vi "HFRR ADV v05.vi"() -> ()   [LabVIEW 2025] (continued)
            n1941 = property on="XY Graph 13" class="XYGraph (strict)"("Y Scale.Display Format:Precision"=u8 0 ("Y Scale.Format & Precision:Precision")) -> ()  [unwired: 2 in, 2 out]
            n1942 = property on="XY Graph 13" class="XYGraph (strict)"("X Scale.Range:Minimum"=0.0, "X Scale.Range:Maximum"=75.0, "Y Scale.Range:Minimum"=0.0, "Y Scale.Range:Maximum"=100.0) -> ()  [unwired: 2 in, 2 out]
          }
        }
        n1943 = case shown="True" "RST CP" {
          frame False {
          }
          frame True {
            n1944 = property on="Sample Temperature" class="XYGraph (strict)"("Y Scale.Display Format:Precision"=u8 2 ("Y Scale.Format & Precision:Precision")) -> ()  [unwired: 2 in, 2 out]
            n1945 = property on="Sample Temperature" class="XYGraph (strict)"("X Scale.Range:Minimum"=0.0, "X Scale.Range:Maximum"=75.0, "Y Scale.Range:Minimum"=58.0, "Y Scale.Range:Maximum"=62.0) -> ()  [unwired: 2 in, 2 out]
          }
        }
        n1946 = case shown="True" "RSTV1 3" {
          frame False {
          }
          frame True {
            n1947 = property on="Air Temperature" class="XYGraph (strict)"("Y Scale.Display Format:Precision"=u8 2 ("Y Scale.Format & Precision:Precision")) -> ()  [unwired: 2 in, 2 out]
            n1948 = property on="Air Temperature" class="XYGraph (strict)"("X Scale.Range:Minimum"=0.0 ("Y Scale.Range:Minimum"), "X Scale.Range:Maximum"=75.0 ("Y Scale.Range:Maximum"), "Y Scale.Range:Minimum"=20.0 ("X Scale.Range:Minimum"), "Y Scale.Range:Maximum"=26.0 ("X Scale.Range:Maximum")) -> ()  [unwired: 2 in, 2 out]
          }
        }
        n1949 = case shown="True" "RSTV1 4" {
          frame False {
          }
          frame True {
            n1950 = property on="Stroke" class="XYGraph (strict)"("Y Scale.Display Format:Precision"=u8 2 ("Y Scale.Format & Precision:Precision")) -> ()  [unwired: 2 in, 2 out]
            n1951 = property on="Stroke" class="XYGraph (strict)"("X Scale.Range:Minimum"=0.0 ("Y Scale.Range:Maximum"), "X Scale.Range:Maximum"=75.0 ("X Scale.Range:Minimum"), "Y Scale.Range:Minimum"=0.98, "Y Scale.Range:Maximum"=1.02) -> ()  [unwired: 2 in, 2 out]
          }
        }
        n1952 = case shown="True" "rstv2" {
          frame False {
          }
          frame True {
            n1953 = property on="Coefficient Of Friction" class="XYGraph (strict)"("Y Scale.Display Format:Precision"=u8 3 ("Y Scale.Format & Precision:Precision")) -> ()  [unwired: 2 in, 2 out]
            n1954 = property on="Coefficient Of Friction" class="XYGraph (strict)"("X Scale.Range:Minimum"=0.0 ("Y Scale.Range:Maximum"), "X Scale.Range:Maximum"=75.0, "Y Scale.Range:Minimum"=0.0, "Y Scale.Range:Maximum"=1.0 ("X Scale.Range:Minimum")) -> ()  [unwired: 2 in, 2 out]
          }
        }
        n1955 = case shown="True" "RST CP 3" {
          frame False {
          }
          frame True {
            n1956 = property on="Air Temp vs Rh" class="XYGraph (strict)"("X Scale.Range:Minimum"=18.0, "X Scale.Range:Maximum"=28.0 ("X Scale.Range:Minimum"), "Y Scale.Range:Minimum"=30.0 ("X Scale.Range:Minimum"), "Y Scale.Range:Maximum"=70.0 ("X Scale.Range:Minimum")) -> ()  [unwired: 2 in, 2 out]
          }
        }
        n1957 = case shown="True" "OPEN 1" {
          frame False {
          }
          frame True {
            (unwired) 0  # existing file
            w2822 = "Choose a datalog file to open"  # prompt
            n1958 = local write "OPEN 1"(FALSE ("OPEN 1")) -> ()
            n1959 = String To Path(string="C:\\LAB-IQ-NXT\\Data\\") -> (path=w2807:path)
            n1960 = File Dialog(6:"*.dgf" ("pattern"), 7:w2822, 11:w2807) -> (0:w2805:errorcluster, 3:w2813:path)  [unwired: 4 in, 2 out]
            n1961 = Unbundle(w2805) -> ()  [unwired: 3 out]
            n1962 = Strip Path(path=w2813) -> (name=w2812:string)  [unwired: 1 out]
            n1963 = Path To String(path=w2813) -> (string=w2808:string)
            "string1" <- w2808
            n1964 = Match Pattern(string=w2812, regular expression=".dgf") -> (before substring=→"String Control":string)  [unwired: 1 in, 3 out]
            n1965 = Match Pattern(string=w2808, regular expression=".dgf" ("substring (\"\")")) -> (before substring=w2818:string)  [unwired: 1 in, 3 out]
            n1966 = Concatenate Strings(w2818, ".duf" ("Substring")) -> (w2814:string)
            n1967 = String To Path(string=w2814) -> (path=w2819:path)
            n1968 = call <vilib>:"Read Characters From File.vi"("file path (dialog if empty)"=w2819, "start of read offset (chars.:0)"=60 ("start of read offset (chars.: 0)")) -> ("character string"=→"String Control 2":string)  [unwired: 4 in, 3 out]
          }
        }
        n1969 = case shown="True" "OPEN 2" {
          frame False {
          }
          frame True {
            (unwired) 0  # existing file
            w2840 = "Choose a datalog file to open"  # prompt
            n1970 = local write "OPEN 2"(FALSE ("OPEN 1")) -> ()
            n1971 = String To Path(string="C:\\LAB-IQ-NXT\\Data\\") -> (path=w2825:path)
            n1972 = File Dialog(6:"*.dgf" ("pattern"), 7:w2840, 11:w2825) -> (0:w2823:errorcluster, 3:w2831:path)  [unwired: 4 in, 2 out]
            n1973 = Unbundle(w2823) -> ()  [unwired: 3 out]
            n1974 = Strip Path(path=w2831) -> (name=w2829:string)  [unwired: 1 out]
            n1975 = Path To String(path=w2831) -> (string=w2826:string)
            "string1 2" <- w2826
            n1976 = Match Pattern(string=w2829, regular expression=".dgf") -> (before substring=→"String Control 3":string)  [unwired: 1 in, 3 out]
            n1977 = Match Pattern(string=w2826, regular expression=".dgf" ("substring (\"\")")) -> (before substring=w2837:string)  [unwired: 1 in, 3 out]
            n1978 = Concatenate Strings(w2837, ".duf" ("Substring")) -> (w2834:string)
            n1979 = String To Path(string=w2834) -> (path=w2832:path)
            n1980 = call <vilib>:"Read Characters From File.vi"("file path (dialog if empty)"=w2832, "start of read offset (chars.:0)"=60 ("start of read offset (chars.: 0)")) -> ("character string"=→"String Control 4":string)  [unwired: 4 in, 3 out]
          }
        }
        n1981 = case shown="True" "OPEN 3" {
          frame False {
          }
          frame True {
            (unwired) 0  # existing file
            w2858 = "Choose a datalog file to open"  # prompt
            n1982 = local write "OPEN 3"(FALSE ("OPEN 1")) -> ()
            n1983 = String To Path(string="C:\\LAB-IQ-NXT\\Data\\") -> (path=w2843:path)
            n1984 = File Dialog(6:"*.dgf" ("pattern"), 7:w2858, 11:w2843) -> (0:w2841:errorcluster, 3:w2849:path)  [unwired: 4 in, 2 out]
            n1985 = Unbundle(w2841) -> ()  [unwired: 3 out]
            n1986 = Strip Path(path=w2849) -> (name=w2847:string)  [unwired: 1 out]
            n1987 = Path To String(path=w2849) -> (string=w2844:string)
            "string1 3" <- w2844
            n1988 = Match Pattern(string=w2847, regular expression=".dgf") -> (before substring=→"String Control 5":string)  [unwired: 1 in, 3 out]
            n1989 = Match Pattern(string=w2844, regular expression=".dgf" ("substring (\"\")")) -> (before substring=w2854:string)  [unwired: 1 in, 3 out]
            n1990 = Concatenate Strings(w2854, ".duf" ("Substring")) -> (w2851:string)
            n1991 = String To Path(string=w2851) -> (path=w2855:path)
            n1992 = call <vilib>:"Read Characters From File.vi"("file path (dialog if empty)"=w2855, "start of read offset (chars.:0)"=60 ("start of read offset (chars.: 0)")) -> ("character string"=→"String Control 6":string)  [unwired: 4 in, 3 out]
          }
        }
        n1993 = case shown="True" "OPEN 4" {
          frame False {
          }
          frame True {
            (unwired) 0  # existing file
            w2876 = "Choose a datalog file to open"  # prompt
            n1994 = local write "OPEN 4"(FALSE ("OPEN 1")) -> ()
            n1995 = String To Path(string="C:\\LAB-IQ-NXT\\Data\\") -> (path=w2861:path)
            n1996 = File Dialog(6:"*.dgf" ("pattern"), 7:w2876, 11:w2861) -> (0:w2859:errorcluster, 3:w2867:path)  [unwired: 4 in, 2 out]
            n1997 = Unbundle(w2859) -> ()  [unwired: 3 out]
            n1998 = Strip Path(path=w2867) -> (name=w2865:string)  [unwired: 1 out]
            n1999 = Path To String(path=w2867) -> (string=w2862:string)
            "string1 4" <- w2862
            n2000 = Match Pattern(string=w2865, regular expression=".dgf") -> (before substring=→"String Control 7":string)  [unwired: 1 in, 3 out]
            n2001 = Match Pattern(string=w2862, regular expression=".dgf" ("substring (\"\")")) -> (before substring=w2872:string)  [unwired: 1 in, 3 out]
            n2002 = Concatenate Strings(w2872, ".duf" ("Substring")) -> (w2869:string)
            n2003 = String To Path(string=w2869) -> (path=w2873:path)
            n2004 = call <vilib>:"Read Characters From File.vi"("file path (dialog if empty)"=w2873, "start of read offset (chars.:0)"=60 ("start of read offset (chars.: 0)")) -> ("character string"=→"String Control 8":string)  [unwired: 4 in, 3 out]
          }
        }
      }
      frame "About" {
        # "Elapsed time\ncof\nstroke\nmean pos\nTemp\nHumidity"
        n2005 = disable-structure shown="Disabled" {
          frame Disabled {
            n2006 = case shown="True" "Export" {
              frame False {
              }
              frame True {
                w2898 = "                                      " ("string")
                w2900 = "\r"
                (unwired) i16 6 ("width (-)")
                w2977 = "\r"
                w2909 = "\r"
                n2007 = local write "Export"(FALSE ("Export")) -> ()
                n2008 = local read "String 29"() -> (w2946:string)
                n2009 = local read "String 34"() -> (w2934:string)
                n2010 = local read "String 35"() -> (w2929:string)
                n2011 = local read "String 37"() -> (w2925:string)
                n2012 = local read "String 36"() -> (w2922:string)
                n2013 = local read "String 38"() -> (w2919:string)
                n2014 = local read "String 39"() -> (w2916:string)
                n2015 = Match Pattern(string=w2946, regular expression=".dwm") -> (before substring=w2942:string)  [unwired: 1 in, 3 out]
                "before substring" <- w2942
                n2016 = local read "S 38"() -> (w2937:string)
                n2017 = local read "S 39"() -> (w2930:string)
                n2018 = local read "Temperature before test 2"() -> (w2966:dbl)
                n2019 = local read "Temperature after test 2"() -> (w2971:dbl)
                n2020 = local read "Humidity before test 2"() -> (w2952:dbl)
                n2021 = local read "Humidity after test 2"() -> (w2967:dbl)
                n2022 = local read "MWSD 2"() -> (w2963:dbl)
                n2023 = local read "WS1.4 2"() -> (w2979:dbl)
                n2024 = local read "HCF 2"() -> (w2975:dbl)
                n2025 = local read "AVP 2"() -> (w2964:dbl)
                n2026 = Concatenate Strings("1," ("string"), w2937) -> (w2936:string)
                n2027 = Concatenate Strings("2," ("string"), w2934) -> (w2933:string)
                n2028 = Concatenate Strings("3," ("string"), w2930) -> (w2932:string)
                n2029 = Concatenate Strings("4," ("string"), w2929) -> (w2928:string)
                n2030 = Concatenate Strings("5," ("string"), w2925) -> (w2926:string)
                n2031 = Concatenate Strings("6," ("string"), w2922) -> (w2923:string)
                n2032 = Concatenate Strings("7," ("string"), w2919) -> (w2920:string)
                n2033 = Concatenate Strings("8," ("string"), w2916) -> (w2917:string)
                n2034 = local read "Sample ID"() -> (w2984:string)
                n2035 = case shown="\"xlx\"" "Select File Type" {
                  tunnel: w2942 -> [w2987 w2989 w2991]
                  tunnel: [w2985 w2990 w2992] -> w2941
                  frame "xlx" {
                    n2036 = Concatenate Strings(w2987, ".xls" ("string")) -> (w2985:string)
                  }
                  frame "csv" {
                    n2037 = Concatenate Strings(w2989, ".csv" ("string")) -> (w2990:string)
                  }
                  frame "txt" {
                    n2038 = Concatenate Strings(w2991, ".txt" ("string")) -> (w2992:string)
                  }
                }
                n2039 = local read "Test Date"() -> (w2983:string)
                n2040 = local read "String 45"() -> (w2897:string)
                n2041 = local read "String 31"() -> (w2982:string)
                n2042 = local read "String 32"() -> (w2981:string)
                n2043 = local read "TITTLE"() -> (w2905:string)
                n2044 = Number To Fractional String(number=w2952, width (-)=i16 6, precision (6)=i16 2) -> (F-format string=w2951:string)  [unwired: 1 in]
                n2045 = Number To Fractional String(number=w2966, width (-)=i16 6, precision (6)=i16 2) -> (F-format string=w2972:string)  [unwired: 1 in]
                n2046 = Number To Fractional String(number=w2967, width (-)=i16 6, precision (6)=i16 2) -> (F-format string=w2965:string)  [unwired: 1 in]
                n2047 = Number To Fractional String(number=w2971, width (-)=i16 6, precision (6)=i16 2) -> (F-format string=w2970:string)  [unwired: 1 in]
                n2048 = Number To Fractional String(number=w2963, width (-)=i16 6, precision (6)=i16 2) -> (F-format string=w2961:string)  [unwired: 1 in]
                n2049 = Number To Fractional String(number=w2964, width (-)=i16 6, precision (6)=i16 2) -> (F-format string=w2962:string)  [unwired: 1 in]
                n2050 = Number To Fractional String(number=w2975, width (-)=i16 6, precision (6)=i16 2) -> (F-format string=w2976:string)  [unwired: 1 in]
                n2051 = Number To Fractional String(number=w2979, precision (6)=i16 2) -> (F-format string=w2980:string)  [unwired: 2 in]
                n2052 = local read "s.NO"() -> (w2899:string)
                n2053 = Concatenate Strings("=" ("string"), w2905) -> (w2904:string)
                n2054 = Concatenate Strings("S.No," ("string"), "                                       Parameters" ("string")) -> (w2910:string)
                n2055 = Concatenate Strings(w2977, w2936, w2951, w2977, w2933, w2972, w2977, w2932, w2965, w2977, w2928, w2970, w2977, w2926, w2961, w2977, w2923, w2962, w2977, w2920, w2976, w2977, w2917, w2980) -> (w2939:string)
                n2056 = Concatenate Strings(w2909, "," ("string"), w2897, w2899, w2898, w2981, w2984, w2898, w2982, w2983, w2909) -> (w2907:string)
                n2057 = local read "Tested by"() -> (w2913:string)
                n2058 = local read "String 33"() -> (w2914:string)
                n2059 = Concatenate Strings("," ("string"), "                                                                             " ("string")) -> (w2902:string)
                n2060 = Concatenate Strings(w2904, w2900, w2907, w2900, w2910, w2939, w2900, w2902, w2914, w2913) -> (→"export":string)
                n2061 = String To Path(string=w2941) -> (path=w2948:path)
                n2062 = local read "export"() -> (w2943:string)
                n2063 = call <vilib>:"Write Characters To File.vi"("append to file? (new file:F)"=FALSE, "character string"=w2943, "file path (dialog if empty)"=w2948) -> ()  [unwired: 2 in, 1 out]
              }
            }
          }
          frame Enabled {
          }
        }
        n2064 = case shown="True" "OK Button 17" {
          frame False {
          }
          frame True {
            (unwired) 0  # existing file
            w3201 = "Choose a datalog file to open"  # prompt
            n2065 = local write "OK Button 17"(FALSE ("OK Button 17")) -> ()
            n2066 = local read "String"() -> (w3196:string)
            n2067 = String To Path(string=w3196) -> (path=w3197:path)
            n2068 = File Dialog(6:"*.duf" ("pattern"), 7:w3201, 11:w3197) -> (0:w3188:errorcluster, 3:w3207:path)  [unwired: 4 in, 2 out]
            n2069 = Unbundle(w3188) -> ()  [unwired: 3 out]
            n2070 = Open/Create/Replace File "Open File"(file path (use dialog)=w3207) -> (refnum out=w3199:refnum<file>)  [unwired: 5 in, 2 out]
            n2071 = Strip Path(path=w3207) -> (name=w3205:string)  [unwired: 1 out]
            n2072 = Path To String(path=w3207) -> (string=w3190:string)
            n2073 = while {
              tunnel: w3199 -> [w3211]
              i -> [w3208]
              stop <- w3209 continue-if-true
              (unwired) TRUE ("line mode (F)")
              n2074 = Read from Text File "Read File"(file (use dialog)=w3211) -> (text=w3210:string)  [unwired: 3 in, 3 out]
              n2075 = local write "Numeric 16"(w3208) -> ()
              n2076 = String Length(string=w3210) -> (length=w3213:i32)
              n2077 = Greater?(x=w3213, y=1) -> (0:w3209:bool)
            }
            n2078 = local write "String 29"(w3190) -> ()
            n2079 = Search and Replace String(input string=w3190, search string=".duf", replace string=".dgf" ("replace string (\"\")")) -> (result string=→"String Indicator 4":string)  [unwired: 5 in, 3 out]
            n2080 = Match Pattern(string=w3205, regular expression=".dwm") -> (before substring=w3189:string)  [unwired: 1 in, 3 out]
            "String Indicator" <- w3189
            n2081 = Match Pattern(string=w3190, regular expression=".dwm" ("substring (\"\")")) -> (before substring=w3191:string)  [unwired: 1 in, 3 out]
            "String Indicator 3" <- w3191
            n2082 = local write "TITTLE 2"(w3189) -> ()
            n2083 = String To Path(string=w3191) -> (path=w3198:path)
            "path" <- w3198
            n2084 = call <vilib>:"Read Characters From File.vi"("file path (dialog if empty)"=w3198, "start of read offset (chars.:0)"=60 ("start of read offset (chars.: 0)")) -> ("character string"=→"String Indicator 2":string)  [unwired: 4 in, 3 out]
          }
        }
        n2085 = case shown="True" "OK Button 16" {
          frame False {
          }
          frame True {
            n2086 = stacked-sequence {
              frame #0 {
                n2087 = local read "Numeric 16"() -> (w3215:i32)
                n2088 = local write "Numeric 10"(w3215) -> ()
              }
              frame #1 {
                n2089 = local read "S.NO"() -> (→"s.NO":string)
                n2090 = local read "String 29"() -> (w3219:string)
                n2091 = String To Path(string=w3219) -> (path=w3218:path)
                n2092 = Open/Create/Replace File "Open File"(file path (use dialog)=w3218) -> (refnum out=w3220:refnum<file>)  [unwired: 5 in, 2 out]
                n2093 = for {
                  N: 16 -> [_]
                  tunnel: w3220 -> [w3227]
                  i -> [w3223]
                  (unwired) TRUE ("line mode (F)")
                  n2094 = Read from Text File "Read File"(file (use dialog)=w3227) -> (text=w3221:string)  [unwired: 3 in, 3 out]
                  n2095 = Match Pattern(string=w3221, regular expression="(") -> (after substring=w3226:string)  [unwired: 1 in, 3 out]
                  n2096 = Match Pattern(string=w3226, regular expression=")") -> (before substring=w3222:string)  [unwired: 1 in, 3 out]
                  n2097 = case shown="1" w3223 {
                    tunnel: w3222 -> [w3228 w3229 _ _ w3230 w3231 w3232 w3234 w3236 w3238 w3240 w3242 w3244 w3246 _]
                    tunnel: w3221 -> [_ _ _ _ _ _ _ _ _ _ _ _ _ _ _]
                    frame 0 {
                      "TITTLE" <- w3228
                    }
                    frame 1 {
                      "Sample ID" <- w3229
                    }
                    frame 2 {
                    }
                    frame 3 {
                    }
                    frame 4 {
                      "Test Date" <- w3230
                    }
                    frame 5 {
                      "Tested by" <- w3231
                    }
                    frame 6 {
                      n2098 = Fract/Exp String To Number(string=w3232) -> (number=→"Humidity before test 2":dbl)  [unwired: 3 in, 1 out]
                    }
                    frame 7 {
                      n2099 = Fract/Exp String To Number(string=w3234) -> (number=→"Temperature before test 2":dbl)  [unwired: 3 in, 1 out]
                    }
                    frame 8 {
                      n2100 = Fract/Exp String To Number(string=w3236) -> (number=→"Humidity after test 2":dbl)  [unwired: 3 in, 1 out]
                    }
                    frame 9 {
                      n2101 = Fract/Exp String To Number(string=w3238) -> (number=→"Temperature after test 2":dbl)  [unwired: 3 in, 1 out]
                    }
                    frame 10 {
                      n2102 = Fract/Exp String To Number(string=w3240) -> (number=→"MWSD 2":dbl)  [unwired: 3 in, 1 out]
                    }
                    frame 11 {
                      n2103 = Fract/Exp String To Number(string=w3242) -> (number=→"AVP 2":dbl)  [unwired: 3 in, 1 out]
                    }
                    frame 12 {
                      n2104 = Fract/Exp String To Number(string=w3244) -> (number=→"HCF 2":dbl)  [unwired: 3 in, 1 out]
                    }
                    frame 13 {
                      n2105 = Fract/Exp String To Number(string=w3246) -> (number=→"WS1.4 2":dbl)  [unwired: 3 in, 1 out]
                    }
                    frame 14, Default {
                    }
                  }
                }
              }
              frame #2 {
              }
            }
            n2106 = local write "OK Button 16"(FALSE ("OK Button 13")) -> ()
          }
        }
        n2107 = call <vilib>:"Query Available Printers.vi"() -> ("system configured printers"=w2890:string[])  [unwired: 9 in, 2 out]
        "System Configured Printers 2" <- w2890
        n2108 = local read "OK Button 16"() -> (w2887:bool)
        n2109 = Index Array(array=w2890, index="Select Printer 3") -> (element=w2892:string)
        "Selected Printer" <- w2892
        n2110 = case shown="True" w2887 {
          frame False {
          }
          frame True {
            n2111 = flat-sequence {
              frame #0 {
              }
              frame #1 {
                n2112 = Wait (ms)(milliseconds to wait=u32 100) -> ()  [unwired: 1 out]
              }
              frame #2 {
                n2113 = local write "OK Button 16"(FALSE ("Print 3")) -> ()
              }
            }
          }
        }
        n2114 = case shown="True" "Print" {
          tunnel: w2892 -> [_ w3184]
          frame False {
          }
          frame True {
            (unwired) i16 6 ("width (-)")
            (unwired) "TESTED BY : "
            (unwired) "TESTED DATE :"
            (unwired) "SAMPLE ID : "
            (unwired) "SAMPLE DESIGN : "
            w3142 = "\r"
            w3159 = "\r"
            # "add image"
            n2115 = local read "Sample ID"() -> (w3132:string)
            n2116 = local read "Tested by"() -> (w3135:string)
            n2117 = local read "String 34"() -> (w3122:string)
            n2118 = local read "String 45"() -> (w3102:string)
            n2119 = local read "String 35"() -> (w3117:string)
            n2120 = local read "String 37"() -> (w3115:string)
            n2121 = local read "String 32"() -> (w3137:string)
            n2122 = local read "String 36"() -> (w3112:string)
            n2123 = local read "String 31"() -> (w3136:string)
            n2124 = local read "Test Date"() -> (w3133:string)
            n2125 = local read "String 33"() -> (w3138:string)
            n2126 = local read "String 38"() -> (w3108:string)
            n2127 = local read "String 39"() -> (w3105:string)
            n2128 = local write "Print"(FALSE ("Print FF")) -> ()
            n2129 = local read "S 39"() -> (w3120:string)
            n2130 = local read "S 38"() -> (w3127:string)
            n2131 = local read "Temperature before test 2"() -> (w3158:dbl)
            n2132 = local read "Temperature after test 2"() -> (w3148:dbl)
            n2133 = local read "Humidity before test 2"() -> (w3173:dbl)
            n2134 = local read "Humidity after test 2"() -> (w3157:dbl)
            n2135 = local read "MWSD 2"() -> (w3162:dbl)
            n2136 = local read "WS1.4 2"() -> (w3140:dbl)
            n2137 = Concatenate Strings("2)" ("string"), w3122) -> (w3123:string)
            n2138 = Concatenate Strings("3)" ("string"), w3120) -> (w3121:string)
            n2139 = Concatenate Strings("1)" ("string"), w3127) -> (w3126:string)
            n2140 = Concatenate Strings("4)" ("string"), w3117) -> (w3118:string)
            n2141 = Concatenate Strings("5)" ("string"), w3115) -> (w3114:string)
            n2142 = Concatenate Strings("6)" ("string"), w3112) -> (w3111:string)
            n2143 = Concatenate Strings("7)" ("string"), w3108) -> (w3109:string)
            n2144 = Concatenate Strings("8)" ("string"), w3105) -> (w3106:string)
            n2145 = local read "HCF 2"() -> (w3144:dbl)
            n2146 = local read "AVP 2"() -> (w3161:dbl)
            n2147 = local read "s.NO"() -> (w3103:string)
            n2148 = call <vilib>:"New Report.vi"("report type"=enum16{"Standard Report", "HTML"}."Standard Report") -> ("report out"=w3182:refnum<class "NI_report.lvclass">, "error out"=w3181:errorcluster)  [unwired: 13 in]
            n2149 = local read "TITTLE"() -> (w3134:string)
            n2150 = Concatenate Strings(w3159, w3102, w3103, w3159, w3137, w3132, w3159, w3136, w3133, w3159, w3138, w3135, w3159) -> (w3152:string)
            "test by" <- w3152
            n2151 = Number To Fractional String(number=w3158, width (-)=i16 6, precision (6)=i16 2) -> (F-format string=w3147:string)  [unwired: 1 in]
            n2152 = Number To Fractional String(number=w3157, width (-)=i16 6, precision (6)=i16 2) -> (F-format string=w3160:string)  [unwired: 1 in]
            n2153 = Number To Fractional String(number=w3173, width (-)=i16 6, precision (6)=i16 2) -> (F-format string=w3178:string)  [unwired: 1 in]
            n2154 = Number To Fractional String(number=w3162, width (-)=i16 6, precision (6)=i16 2) -> (F-format string=w3164:string)  [unwired: 1 in]
            n2155 = Number To Fractional String(number=w3148, width (-)=i16 6, precision (6)=i16 2) -> (F-format string=w3149:string)  [unwired: 1 in]
            n2156 = Number To Fractional String(number=w3161, width (-)=i16 6, precision (6)=i16 2) -> (F-format string=w3163:string)  [unwired: 1 in]
            n2157 = Number To Fractional String(number=w3144, width (-)=i16 6, precision (6)=i16 2) -> (F-format string=w3143:string)  [unwired: 1 in]
            n2158 = Number To Fractional String(number=w3140, precision (6)=i16 2) -> (F-format string=w3139:string)  [unwired: 2 in]
            n2159 = call-dynamic "Set Report Header Text.vi"("report in"=w3182, "center header text"=w3134, "error in (no error)"=w3181) -> ("report out"=w3153:refnum<class "NI_report.lvclass">, "error out"=w3154:errorcluster)  [unwired: 11 in]
            n2160 = Concatenate Strings(w3142, w3126, w3178, w3142, w3123, w3147, w3142, w3121, w3160, w3142, w3118, w3149, w3142, w3114, w3164, w3142, w3111, w3163, w3142, w3109, w3143, w3142, w3106, w3139) -> (w3130:string)
            "export 2" <- w3130
            n2161 = call-poly <vilib>:"Append Report Text.vi"("report in"=w3153, "text"=w3152, "error in (no error)"=w3154) -> ("report out"=w3156:refnum<class "NI_report.lvclass">, "error out"=w3155:errorcluster)  [unwired: 9 in, 2 out]
            n2162 = local read "test by"() -> (w3129:string)
            n2163 = local read "TITTLE"() -> (w3131:string)
            n2164 = call-poly <vilib>:"Append Report Text.vi"("report in"=w3156, "error in (no error)"=w3155) -> ("report out"=w3177:refnum<class "NI_report.lvclass">, "error out"=w3175:errorcluster)  [unwired: 10 in, 2 out]
            n2165 = Concatenate Strings(w3131, w3130, w3129) -> (→"output":string)
            n2166 = call-poly <vilib>:"Append Report Text.vi"("report in"=w3177, "text"=w3130, "error in (no error)"=w3175) -> ("report out"=w3176:refnum<class "NI_report.lvclass">, "error out"=w3174:errorcluster)  [unwired: 9 in, 2 out]
            n2167 = call-dynamic "Print Report.vi"("report in"=w3176, "printer name (default)"=w3184, "error in (no error)"=w3174) -> ("report out"=w3186:refnum<class "NI_report.lvclass">, "error out"=w3187:errorcluster)  [unwired: 11 in]
            n2168 = call-dynamic "Dispose Report.vi"("report in"=w3186, "error in (no error)"=w3187) -> ()  [unwired: 13 in, 1 out]
          }
        }
        n2169 = case shown="True" "Print 2" {
          frame False {
          }
          frame True {
            n2170 = flat-sequence {
              frame #0 {
                n2171 = local read "s.NO"() -> (→"s.NO 2":string)
                n2172 = Wait (ms)(milliseconds to wait=u32 20) -> ()  [unwired: 1 out]
                n2173 = local read "Sample ID  3"() -> (→"Sample ID  6":string)
                n2174 = local read "Sample ID  4"() -> (→"Sample ID  7":string)
                n2175 = local read "Sample ID"() -> (→"Sample ID  2":string)
                n2176 = local read "Tested by"() -> (→"Tested by 2":string)
                n2177 = local read "Test Date"() -> (→"Test Date 2":string)
                n2178 = local read "Humidity after test 3"() -> (→"Humidity after test 4":dbl)
                n2179 = local read "Ref A Test Date :"() -> (→"TITTLE 4":string)
                n2180 = local read "Temperature before test 3"() -> (w3009:dbl)
                n2181 = local read "Temperature before test 3"() -> (→"Temperature after test 5":dbl)
                n2182 = local read "Temperature after test 3"() -> (→"Temperature after test 4":dbl)
                n2183 = local read "Humidity before test 3"() -> (→"Humidity before test 4":dbl)
                n2184 = local write "Temperature before test 3"(w3009) -> ()
                n2185 = local read "image data"() -> (w3000:T11)
                n2186 = String To Path(string="C:\\LAB-IQ-NXT\\im\\Temp_resized.jpg") -> (path=w3001:path)
                "path 2" <- w3001
                n2187 = call <vilib>:"Write JPEG File.vi"("image data"=w3000, "path to JPEG file"=w3001) -> ()  [unwired: 8 in, 2 out]
                "Ref A Test Date :" <- "Ref A Test Date :"
                "Ref B Test Date :" <- "Ref B Test Date :"
                "Ref B Scar Value :" <- "Ref B Scar Value :"
                "Ref A Scar Value :" <- "Ref A Scar Value :"
              }
              frame #1 {
                (unwired) HTML_Report_Image_Alignment."MIDDLE" ("alignment (default)")
                w3037 = u16 0 items=["portrait", "landscape"] ("orientation (portrait)")
                (unwired) HTML_Report_Image_Alignment."ABSMIDDLE" ("alignment (default)")
                (unwired) "TESTED BY : "
                (unwired) "TESTED DATE :"
                (unwired) "SAMPLE ID : "
                (unwired) "SAMPLE DESIGN : "
                w3070 = "\r"
                # "add image"
                n2188 = Wait (ms)(milliseconds to wait=u32 20) -> ()  [unwired: 1 out]
                n2189 = local read "Sample ID  2"() -> (w3063:string)
                n2190 = local read "Wear Scar X"() -> (w3035:dbl)
                "Length ( microns ) 2" <- w3035
                n2191 = local read "Wear Scar Y"() -> (w3034:dbl)
                "Wear Scar Y ( microns ) :" <- w3034
                n2192 = local read "Test Date 2"() -> (w3064:string)
                n2193 = local read "Tested by 2"() -> (w3065:string)
                n2194 = local read "String 46"() -> (w3061:string)
                n2195 = local read "String 48"() -> (w3067:string)
                n2196 = local read "String 47"() -> (w3066:string)
                n2197 = local read "String 49"() -> (w3068:string)
                n2198 = local read "String 10"() -> (w3021:string)
                n2199 = local read "s.NO 2"() -> (w3062:string)
                n2200 = Add(x=w3035, y=w3034) -> (x+y=w3033:dbl)
                n2201 = call <vilib>:"New Report.vi"("report type"=enum16{"Standard Report", "HTML"}."HTML") -> ("report out"=w3041:refnum<class "NI_report.lvclass">, "error out"=w3039:errorcluster)  [unwired: 13 in]
                n2202 = Concatenate Strings(w3070, w3061, w3062, w3070, w3067, w3063, w3070, w3066, w3064, w3070, w3068, w3065, w3070) -> (→"test by 2":string)
                n2203 = Concatenate Strings("C:\\LAB-IQ-NXT\\Data\\" ("string"), w3021, ".jpg" ("string")) -> ()  [unwired: 1 out]
                n2204 = Divide(x=w3033, y=2.0) -> (x/y=→"Mean Wear ( microns) :":dbl)
                n2205 = call-dynamic "Set Report Orientation.vi"("report in"=w3041, "orientation (portrait)"=w3037, "error in (no error)"=w3039) -> ("report out"=w3040:refnum<class "NI_report.lvclass">, "error out"=w3038:errorcluster)  [unwired: 11 in]
                n2206 = for {
                  N: 5 -> [_]
                  tunnel: w3040 -> [w3091]
                  tunnel: [w3090] -> w3019
                  tunnel: w3038 -> [w3089]
                  tunnel: [w3088] -> w3018
                  n2207 = call-dynamic "Set Report Tab Width.vi"("report in"=w3091, "error in (no error)"=w3089) -> ("report out"=w3090:refnum<class "NI_report.lvclass">, "error out"=w3088:errorcluster)  [unwired: 12 in]
                }
                n2208 = local read "TITTLE"() -> (w3036:string)
                n2209 = call-dynamic "Set Report Header Text.vi"("report in"=w3019, "center header text"=w3036, "error in (no error)"=w3018) -> ("report out"=w3057:refnum<class "NI_report.lvclass">, "error out"=w3056:errorcluster)  [unwired: 11 in]
                n2210 = for {
                  N: 1 -> [_]
                  tunnel: [w3095] -> w3043
                  tunnel: [w3094] -> w3042
                  tunnel: w3057 -> [w3093]
                  tunnel: w3056 -> [w3092]
                  n2211 = call-dynamic "New Report Line.vi"("report in"=w3093, "error in (no error)"=w3092) -> ("report out"=w3095:refnum<class "NI_report.lvclass">, "error out"=w3094:errorcluster)  [unwired: 12 in]
                }
                n2212 = for {
                  N: 2 -> [_]
                  tunnel: [w3087] -> w3049
                  tunnel: [w3086] -> w3048
                  tunnel: w3043 -> [w3085]
                  tunnel: w3042 -> [w3084]
                  n2213 = call-dynamic "New Report Line.vi"("report in"=w3085, "error in (no error)"=w3084) -> ("report out"=w3087:refnum<class "NI_report.lvclass">, "error out"=w3086:errorcluster)  [unwired: 12 in]
                }
                n2214 = for {
                  N: 25 -> [_]
                  tunnel: w3049 -> [w3083]
                  tunnel: w3048 -> [w3081]
                  tunnel: [w3082] -> w3052
                  tunnel: [w3080] -> w3051
                  n2215 = call-dynamic "Set Report Tab Width.vi"("report in"=w3083, "error in (no error)"=w3081) -> ("report out"=w3082:refnum<class "NI_report.lvclass">, "error out"=w3080:errorcluster)  [unwired: 12 in]
                }
                n2216 = control-ref of="Tab Control 9"() -> (w3047:refnum<vi>)
                n2217 = call-dynamic "Append Control Image to Report.vi"("report in"=w3052, "alignment (default)"=HTML_Report_Image_Alignment."ABSMIDDLE", "ctrl reference"=w3047, "error in (no error)"=w3051) -> ("report out"=w3046:refnum<class "NI_report.lvclass">, "error out"=w3045:errorcluster)  [unwired: 8 in, 2 out]
                n2218 = for {
                  N: 3 -> [_]
                  tunnel: [w3079] -> w3030
                  tunnel: [w3078] -> w3029
                  tunnel: w3046 -> [w3077]
                  tunnel: w3045 -> [w3076]
                  n2219 = call-dynamic "New Report Line.vi"("report in"=w3077, "error in (no error)"=w3076) -> ("report out"=w3079:refnum<class "NI_report.lvclass">, "error out"=w3078:errorcluster)  [unwired: 12 in]
                }
                n2220 = for {
                  N: 100 -> [_]
                  tunnel: w3030 -> [w3075]
                  tunnel: w3029 -> [w3073]
                  tunnel: [w3074] -> w3026
                  tunnel: [w3072] -> w3024
                  n2221 = call-dynamic "Set Report Tab Width.vi"("report in"=w3075, "error in (no error)"=w3073) -> ("report out"=w3074:refnum<class "NI_report.lvclass">, "error out"=w3072:errorcluster)  [unwired: 12 in]
                }
                n2222 = String To Path(string="C:\\LAB-IQ-NXT\\im\\Temp_resized.jpg") -> (path=w3016:path)
                n2223 = call-poly <vilib>:"Append Image to Report.vi"("report in"=w3026, "path or URL of image"=w3016, "error in (no error)"=w3024) -> ("report out"=w3025:refnum<class "NI_report.lvclass">, "error out"=w3023:errorcluster)  [unwired: 9 in, 2 out]
                n2224 = call-poly <vilib>:"Open HTML Report in Browser.vi"("report in"=w3025, "error in (no error)"=w3023) -> ("report out"=w3060:refnum<class "NI_report.lvclass">, "error out"=w3059:errorcluster)  [unwired: 11 in, 1 out]
                n2225 = call-dynamic "Dispose Report.vi"("report in"=w3060, "error in (no error)"=w3059) -> ()  [unwired: 13 in, 1 out]
              }
              frame #2 {
              }
              frame #3 {
                n2226 = disable-structure shown="Disabled" {
                  frame Disabled {
                    n2227 = local read "String 10"() -> (w3100:string)
                    n2228 = Concatenate Strings("C:\\LAB-IQ-NXT\\Data\\" ("string"), w3100, ".jpg" ("string")) -> (w3098:string)
                    n2229 = String To Path(string=w3098) -> (path=w3097:path)
                    n2230 = Delete(path (use dialog)=w3097) -> ()  [unwired: 4 in, 3 out]
                  }
                  frame Enabled {
                  }
                }
                n2231 = local write "Print 2"(FALSE ("Print")) -> ()
              }
            }
          }
        }
      }
    }
    n2232 = property on="SetTemp" class="DigNum (strict)"("Disabled"=w1100) -> ()  [unwired: 2 in, 2 out]
    n2233 = Multiply(x=w1089, y=w1091) -> (x*y=w1090:dbl)
    n2234 = local read "MWSD"() -> (w1088:dbl)
    n2235 = Add(x=w1090, y=w1088) -> (x+y=→"WS1.4":dbl)
    n2236 = Wait (ms)(milliseconds to wait=u32 50) -> ()  [unwired: 1 out]
    n2237 = Wait (ms)(milliseconds to wait=u32 50) -> ()  [unwired: 1 out]
    n2238 = local read "Quit"() -> (w1087:bool)
  }
  n2239 = VISA Close(VISA resource name=w36, error in (no error)=w35) -> (error out=w33:errorcluster)
  n2240 = VISA Close(VISA resource name=w16, error in (no error)=w15) -> ()  [unwired: 1 out]
  n2241 = call <vilib>:"Clear Errors.vi"("error in (no error)"=w33) -> ()  [unwired: 5 in, 2 out]
  n2242 = Or(x=w23, y=w22) -> (x .or. y?=w24:bool)
  n2243 = while {
    tunnel: [w3248] -> w29
    shift-right: [w3286] -> _
    shift-left: "" -> [w3274]
    tunnel: [w3262] -> _
    i -> [w3262]
    stop <- w3248 stop-if-true
    w3288 = ";" ("string")
    n2244 = local read "start en"() -> (w3307:bool)
    n2245 = And(x="st enable", y=w3307) -> (x .and. y?=w3308:bool)
    n2246 = local read "ACQUIRE 3"() -> (w3251:bool)
    n2247 = local read "Elapsed time"() -> (w3270:dbl)
    n2248 = case shown="True" w3308 {
      tunnel: "st enable" -> [w3372 w3373]
      tunnel: [w3372 w3373] -> w3252
      frame False {
      }
      frame True {
        n2249 = local write "start en"(FALSE ("start en")) -> ()
      }
    }
    n2250 = Wait (ms)(milliseconds to wait=u32 80) -> ()  [unwired: 1 out]
    n2251 = local read "Stroke"() -> (w3261:dbl)
    n2252 = Greater?(x=w3270, y=0.1) -> (0:w3268:bool)
    n2253 = Or(x=w3252, y=w3251) -> (x .or. y?=w3253:bool)
    n2254 = case shown="True" "ACQUIRE 2" {
      frame False {
      }
      frame True {
        n2255 = call "Elapsed Time13"() -> ("Time has Elapsed"=w3315:bool)  [unwired: 12 in, 7 out]
        n2256 = case shown="True" w3315 {
          frame False {
          }
          frame True {
            n2257 = local write "ACQUIRE 2"(FALSE ("ACQUIRE 2")) -> ()
            n2258 = local write "ACQUIRE 3"(FALSE ("ACQUIRE 2")) -> ()
          }
        }
        n2259 = local write "ACQUIRE 3"(TRUE ("ACQUIRE 2")) -> ()
      }
    }
    n2260 = case shown="True" w3253 {
      tunnel: w3261 -> [_ w3395]
      tunnel: [w3375 _] -> w3305
      tunnel: w3268 -> [_ _]
      tunnel: w3251 -> [_ w3382]
      frame False {
        w3375 = TRUE ("PID Rst")
        n2261 = local read "stop cmd"() -> (w3376:bool)
        n2262 = case shown="True" w3376 {
          frame False {
          }
          frame True {
            n2263 = local write "stop cmd"(FALSE ("stop cmd")) -> ()
          }
        }
        n2264 = local write "PID Rst"(TRUE ("PID Rst")) -> ()
        "start en" <- w3375
      }
      frame True {
        w3402 = cluster{"output high":dbl, "output low":dbl} {"output high"=600.0, "output low"=-600.0} ("output range")
        n2265 = local read "STROKE GAIN :"() -> (w3387:dbl)
        n2266 = call "Elapsed Time6"("Reset"="PID Rst", "Auto Reset"=FALSE) -> ("Time has Elapsed"=w3396:bool)  [unwired: 10 in, 7 out]
        n2267 = Multiply(x="Set Strk", y=w3387) -> (x*y=w3380:dbl)
        n2268 = case shown="False" w3396 {
          tunnel: [w3407 w3408] -> w3399
          tunnel: "Set Strk" -> [w3407 _]
          tunnel: w3395 -> [_ w3408]
          frame False {
          }
          frame True {
          }
        }
        n2269 = Multiply(x=w3380, y=1.0) -> (x*y=w3379:dbl)
        n2270 = Select(t=T8 {"Proportional Gain (Kc)"=0.0, "Integral Time (Ti, min)"=0.02, "Derivative Time (Td, min)"=0.0} ("Stroke PID Gains"), s=w3382, f="Stroke PID Gains") -> (s? t:f=w3383:T8)
        n2271 = Not(x=w3396) -> (.not. x?=w3394:bool)
        n2272 = call-poly <vilib>:"PID.vi"("reinitialize? (F)"=w3394, "output range"=w3402, "PID gains"=w3383, "process variable"=w3399, "setpoint"="Set Strk") -> ("output"=w3393:dbl)  [unwired: 5 in, 1 out]
        "Slide 5" <- w3393
        n2273 = Select(t=w3393, s=w3396, f=0.0) -> (s? t:f=w3397:dbl)
        n2274 = flat-sequence {
          tunnel: w3397 -> [_]
          frame #0 {
            n2275 = local write "PID Rst"(FALSE ("PID Rst")) -> ()
          }
        }
        n2276 = Add(x=w3379, y=w3397) -> (x+y=w3392:dbl)
        n2277 = Unbundle(w3402) -> ("output high"=w3401:dbl, "output low"=w3400:dbl)
        n2278 = To Word Integer(number=w3392) -> (16bit integer=w3389:i16)
        n2279 = property on="Slide 5" class="Slide (strict)"("Scale.Range:Minimum"=w3400, "Scale.Range:Maximum"=w3401) -> ()  [unwired: 2 in, 2 out]
        n2280 = In Range and Coerce(upper limit=4095.0 ("f"), x=w3389, lower limit=100.0 ("f")) -> (coerced(x)=w3386:dbl)  [unwired: 1 out]
        "PID Out" <- w3386
        n2281 = Number To Decimal String(number=w3386) -> (decimal integer string=→"st gain":string)  [unwired: 1 in]
        "stop cmd" <- TRUE ("Auto Reset")
      }
    }
    n2282 = flat-sequence {
      frame #0 {
        n2283 = local read "CH-POWER +"() -> (w3319:u16)
        n2284 = local read "CH-POWER -"() -> (w3320:u16)
        n2285 = case shown="1" w3320 {
          tunnel: "PWR" -> [w3321 w3322 w3323 w3324 w3325 w3326 w3327 w3328]
          frame 0, Default {
            n2286 = local write "Do 0"(w3321) -> ()
          }
          frame 1 {
            n2287 = local write "Do 1"(w3322) -> ()
          }
          frame 2 {
            n2288 = local write "Do 2"(w3323) -> ()
          }
          frame 3 {
            n2289 = local write "Do 3"(w3324) -> ()
          }
          frame 4 {
            n2290 = local write "Do 4"(w3325) -> ()
          }
          frame 5 {
            n2291 = local write "Do 5"(w3326) -> ()
          }
          frame 6 {
            n2292 = local write "Do 6"(w3327) -> ()
          }
          frame 7 {
            n2293 = local write "Do 7"(w3328) -> ()
          }
        }
        n2294 = case shown="1" w3319 {
          tunnel: "PWR" -> [w3329 w3330 w3331 w3332 w3333 w3334 w3335 w3336]
          frame 0, Default {
            n2295 = local write "Do 0"(w3329) -> ()
          }
          frame 1 {
            n2296 = local write "Do 1"(w3330) -> ()
          }
          frame 2 {
            n2297 = local write "Do 2"(w3331) -> ()
          }
          frame 3 {
            n2298 = local write "Do 3"(w3332) -> ()
          }
          frame 4 {
            n2299 = local write "Do 4"(w3333) -> ()
          }
          frame 5 {
            n2300 = local write "Do 5"(w3334) -> ()
          }
          frame 6 {
            n2301 = local write "Do 6"(w3335) -> ()
          }
          frame 7 {
            n2302 = local write "Do 7"(w3336) -> ()
          }
        }
      }
    }
    n2303 = local read "RUN"() -> (w3259:bool)
    n2304 = Or(x=w3259, y="ACQUIRE 3") -> (x .or. y?=w3258:bool)
    n2305 = local read "Set Hz"() -> (w3276:dbl)
    n2306 = Select(t=w3276, s=w3258, f=0.0) -> (s? t:f=w3275:dbl)
    n2307 = local read "st gain"() -> (w3279:string)
    n2308 = local read "DO"() -> (w3280:string)
    n2309 = case shown="True" "Boolean 10" {
      frame False {
      }
      frame True {
        n2310 = local write "Tab Control 8"(enum32{"setup", "calibrate"}."calibrate" ("Tab Control 8")) -> ()
        n2311 = local write "Boolean 10"(FALSE ("Boolean 10")) -> ()
      }
    }
    n2312 = Number To Decimal String(number=w3275) -> (decimal integer string=w3278:string)  [unwired: 1 in]
    n2313 = case shown="True" "Boolean 11" {
      frame False {
      }
      frame True {
        n2314 = local write "Tab Control 8"(enum32{"setup", "calibrate"}."setup" ("Tab Control 8")) -> ()
        n2315 = local write "Boolean 11"(FALSE ("Boolean 11")) -> ()
      }
    }
    n2316 = String Length(string=w3279) -> (length=w3294:i32)
    n2317 = String Length(string=w3280) -> (length=w3282:i32)
    n2318 = String Length(string=w3278) -> (length=w3295:i32)
    n2319 = Subtract(x=4.0, y=w3294) -> (x-y=w3291:dbl)
    n2320 = Subtract(x=3.0, y=w3282) -> (x-y=w3285:dbl)
    n2321 = flat-sequence {
      tunnel: w3305 -> [_]
      frame #0 {
        n2322 = Build Array("Do 0", "Do 1", "Do 2", "Do 3", "Do 4", "Do 5", "Do 6", "Do 7") -> (w3363:bool[])
        n2323 = Boolean Array To Number(Boolean array=w3363) -> (number=w3361:u32)
        n2324 = Add(x=w3361, y=u32 0) -> (x+y=w3359:u32)
        n2325 = Number To Decimal String(number=w3359) -> (decimal integer string=→"DO":string)  [unwired: 1 in]
      }
    }
    n2326 = Subtract(x=3.0, y=w3295) -> (x-y=w3296:dbl)
    n2327 = Replace Substring(3:w3291, 4:w3279, 5:"0000" ("string")) -> (1:w3289:string)  [unwired: 1 in, 1 out]
    n2328 = Replace Substring(3:w3285, 4:w3280, 5:"000" ("string")) -> (1:w3281:string)  [unwired: 1 in, 1 out]
    n2329 = Replace Substring(3:w3296, 4:w3278, 5:"000" ("string")) -> (1:w3290:string)  [unwired: 1 in, 1 out]
    n2330 = Concatenate Strings("*" ("string"), w3290, w3288, w3289, w3288, w3281, "$" ("string")) -> (w3286:string)
    "Stroke_send_Val" <- w3286
    n2331 = local read "RUN"() -> (w3256:bool)
    n2332 = local read "ACQUIRE 3"() -> (w3255:bool)
    n2333 = local read "send"() -> (w3272:bool)
    n2334 = Not Equal?(x=w3274, y=w3286) -> (x != y?=w3287:bool)
    n2335 = Or(x=w3256, y=w3255) -> (x .or. y?=w3254:bool)
    n2336 = And(x=w3272, y=w3254) -> (x .and. y?=w3271:bool)
    n2337 = Or(x=w3287, y=w3271) -> (x .or. y?=w3265:bool)
    n2338 = case shown="False" w3254 {
      frame False {
        "send" <- TRUE ("send")
      }
      frame True {
      }
    }
    n2339 = call "Elapsed Time4"("Time Target (s)"=0.5) -> ("Time has Elapsed"=w3263:bool)  [unwired: 11 in, 7 out]
    n2340 = local read "Din"() -> (w3304:u8[])
    n2341 = Or(x=w3263, y=w3265) -> (x .or. y?=w3264:bool)
    n2342 = local read "Quit"() -> (w3248:bool)
    n2343 = Index Array(array=w3304, index=0) -> (element=w3302:u8)
    n2344 = case shown="True" w3264 {
      tunnel: w3286 -> [_ w3340]
      frame False {
      }
      frame True {
        n2345 = local read "Due Com"() -> (w3341:string[])
        n2346 = Build Array (concatenate)(w3341, w3340) -> (→"Due Com":string[])
        n2347 = local write "send"(FALSE ("send")) -> ()
      }
    }
    n2348 = Number To Boolean Array(number=w3302) -> (Boolean array=w3301:bool[])
    n2349 = Array Size(array=w3301) -> (size(s)=w3300:i32)
    n2350 = Greater Than 0?(x=w3300) -> (x > 0?=w3299:bool)
    n2351 = case shown="True" w3299 {
      tunnel: w3301 -> [_ w3355]
      frame False {
      }
      frame True {
        n2352 = Index Array(array=w3355, index #1=0 ("index"), index #2=1 ("index"), index #3=2 ("index"), index #4=3 ("index"), index #5=4 ("index"), index #6=5 ("index"), index #7=6 ("index"), index #8=7 ("index")) -> (element #1=→"DI 0":bool, element #2=→"DI 1":bool, element #3=→"DI 2":bool, element #4=→"DI 3":bool, element #5=→"DI 4":bool, element #6=→"DI 5":bool, element #7=→"DI 6":bool, element #8=→"DI 7":bool)
      }
    }
  }
  n2353 = Or(x=w19, y=w24) -> (x .or. y?=w31:bool)
  n2354 = control-ref of="new picture"() -> ()  [unwired: 1 out]
  n2355 = Or(x=w38, y=w31) -> (x .or. y?=w28:bool)
  n2356 = Or(x=w28, y=w29) -> (x .or. y?=w20:bool)
  n2357 = while {
    tunnel: [w3410] -> w42
    tunnel: [w3411] -> _
    i -> [w3411]
    stop <- w3410 stop-if-true
    n2358 = local read "PID-out"() -> (w3412:dbl)
    "Horizontal Slider Control" <- w3412
    n2359 = Greater Or Equal?(x=w3412, y=2.0) -> (x >= y?=w3413:bool)
    n2360 = flat-sequence {
      tunnel: w3413 -> [w3421]
      tunnel: w3412 -> [w3424]
      tunnel: [w3422] -> w3419
      tunnel: [w3420] -> w3418
      tunnel: [w3440] -> w3417
      tunnel: w3419 -> [w3440]
      tunnel: w3418 -> [w3437]
      tunnel: [w3437] -> w3416
      tunnel: w3417 -> [w3442]
      tunnel: [w3441] -> w3415
      tunnel: w3416 -> [w3441]
      tunnel: w3415 -> [w3456]
      frame #0 {
        n2361 = case shown="True" w3421 {
          selector: w3421 -> [w3426 _]
          frame False {
            n2362 = local write "HEATER"(w3426) -> ()
          }
          frame True {
            w3428 = TRUE ("data")
            n2363 = local read "CH-HEATER"() -> (w3427:u16)
            n2364 = case shown="2" w3427 {
              tunnel: w3428 -> [w3429 w3430 w3431 w3432 w3433 w3434 w3435 w3436]
              frame 0, Default {
                n2365 = local write "Do 0"(w3429) -> ()
              }
              frame 1 {
                n2366 = local write "Do 1"(w3430) -> ()
              }
              frame 2 {
                n2367 = local write "Do 2"(w3431) -> ()
              }
              frame 3 {
                n2368 = local write "Do 3"(w3432) -> ()
              }
              frame 4 {
                n2369 = local write "Do 4"(w3433) -> ()
              }
              frame 5 {
                n2370 = local write "Do 5"(w3434) -> ()
              }
              frame 6 {
                n2371 = local write "Do 6"(w3435) -> ()
              }
              frame 7 {
                n2372 = local write "Do 7"(w3436) -> ()
              }
            }
            "HEATER" <- w3428
          }
        }
        n2373 = Select(t=w3424, s=w3421, f=0.0) -> (s? t:f=w3420:dbl)
        n2374 = Greater Or Equal?(x=w3424, y=97.0) -> (x >= y?=w3422:bool)
      }
      frame #1 {
        n2375 = Multiply(x=w3437, y=5.0) -> (x*y=w3439:dbl)
        n2376 = Wait (ms)(milliseconds to wait=w3439) -> ()  [unwired: 1 out]
      }
      frame #2 {
        n2377 = case shown="False" w3442 {
          frame False {
            w3443 = FALSE ("data")
            n2378 = local read "CH-HEATER"() -> (w3444:u16)
            n2379 = case shown="4" w3444 {
              tunnel: w3443 -> [w3445 w3446 w3447 w3448 w3449 w3450 w3451 w3452]
              frame 0, Default {
                n2380 = local write "Do 0"(w3445) -> ()
              }
              frame 1 {
                n2381 = local write "Do 1"(w3446) -> ()
              }
              frame 2 {
                n2382 = local write "Do 2"(w3447) -> ()
              }
              frame 3 {
                n2383 = local write "Do 3"(w3448) -> ()
              }
              frame 4 {
                n2384 = local write "Do 4"(w3449) -> ()
              }
              frame 5 {
                n2385 = local write "Do 5"(w3450) -> ()
              }
              frame 6 {
                n2386 = local write "Do 6"(w3451) -> ()
              }
              frame 7 {
                n2387 = local write "Do 7"(w3452) -> ()
              }
            }
            n2388 = local write "HEATER"(w3443) -> ()
          }
          frame True {
          }
        }
      }
      frame #3 {
        n2389 = Subtract(x=100, y=w3456) -> (x-y=w3455:dbl)
        n2390 = Multiply(x=w3455, y=5.0) -> (x*y=w3453:dbl)
        n2391 = Wait (ms)(milliseconds to wait=w3453) -> ()  [unwired: 1 out]
      }
    }
    n2392 = local read "Quit"() -> (w3410:bool)
  }
  n2393 = Or(x=w42, y=w20) -> (x .or. y?=w41:bool)
  n2394 = while {
    tunnel: [w3458] -> w37
    i -> [w3465]
    stop <- w3458 stop-if-true
    n2395 = local read "Quit"() -> (w3458:bool)
    n2396 = Equal To 0?(x=w3465) -> (x = 0?=w3463:bool)
    n2397 = call "Elapsed Time3"("Time Target (s)"=45.0, "Auto Reset"=TRUE) -> ("Time has Elapsed"=w3462:bool)  [unwired: 10 in, 7 out]
    n2398 = Wait (ms)(milliseconds to wait=u32 50) -> ()  [unwired: 1 out]
    n2399 = Or(x=w3462, y=w3463) -> (x .or. y?=w3464:bool)
    n2400 = case shown="True" w3464 {
      frame False {
      }
      frame True {
        n2401 = call <vilib>:"System Exec.vi"("run minimized? (F)"=TRUE, "error in (no error)"="error in (no error)", "command line"="powercfg.exe -change -monitor-timeout-ac 0") -> ("error out"=w3476:errorcluster)  [unwired: 5 in, 3 out]
        n2402 = call <vilib>:"System Exec.vi"("run minimized? (F)"=TRUE, "error in (no error)"=w3476, "command line"="powercfg.exe -change -disk-timeout-ac 0") -> ("error out"=w3475:errorcluster)  [unwired: 5 in, 3 out]
        n2403 = call <vilib>:"System Exec.vi"("run minimized? (F)"=TRUE, "error in (no error)"=w3475, "command line"="powercfg.exe -change -standby-timeout-ac 0") -> ("error out"=w3474:errorcluster)  [unwired: 5 in, 3 out]
        n2404 = call <vilib>:"System Exec.vi"("run minimized? (F)"=TRUE, "error in (no error)"=w3474, "command line"="powercfg.exe -change -hibernate-timeout-ac 0") -> ("error out"=w3473:errorcluster)  [unwired: 5 in, 3 out]
        n2405 = call <vilib>:"Simple Error Handler.vi"("error in (no error)"=w3473) -> ("error out"=w3479:errorcluster)  [unwired: 4 in, 4 out]
        n2406 = call <vilib>:"Clear Errors.vi"("error in (no error)"=w3479) -> ("error out"=→"error out":errorcluster)  [unwired: 5 in, 1 out]
      }
    }
  }
  n2407 = Compound Arithmetic op=OR(w40, w41, w37) -> (w39:bool)
  n2408 = flat-sequence {
    tunnel: w39 -> [_]
    frame #0 {
    }
    frame #1 {
      n2409 = Quit LabVIEW(quit? (T)=TRUE) -> ()
      n2410 = local write "Quit"(FALSE ("EXIT")) -> ()
    }
  }
  n2411 = property on="Heater Button" class="Bool (strict)"("Visible"=TRUE) -> ()  [unwired: 2 in, 2 out]
  n2412 = disable-structure shown="Disabled" {
    disable-tunnel: _ -> [w3486 _]
    disable-tunnel: _ -> [w3483 _]
    disable-tunnel: _ -> [w3484 _]
    frame Disabled {
      n2413 = disable-structure shown="Disabled" {
        disable-tunnel: [w3493 _] -> w3485
        frame Disabled {
          n2414 = while {
            shift-right: [w3535] -> w3491
            shift-left: errorcluster {"status"=TRUE, "code"=0, "source"="Init"} ("error out") -> [w3500]
            shift-right: [w3534] -> w3490
            shift-left: _ -> [w3501]
            shift-right: [w3533] -> _
            shift-left: "" -> [w3532]
            tunnel: [w3494] -> w3493
            shift-right: ["Set Rh"] -> _
            shift-left: 0.0 ("Set Rh") -> [w3526]
            tunnel: [w3503] -> _
            i -> [w3503]
            stop <- w3494 stop-if-true
            n2415 = flat-sequence {
              tunnel: w3500 -> [w3538]
              tunnel: [w3538] -> w3499
              frame #0 {
